vi "MeasurementControl - Main.vi"() -> ()   [LabVIEW 2014]
doc: "This VI provides control and an interface the various instruments used to collect data in the CLTC measurement lab. It is built based on the queued message handler template. It functions by sending commands to the queues of the various instrument VIs that are dynamically launched for a particular test."
uses:
  controls/Tab Control.ctl
  controls/Instrument Control Switches.ctl
  Timing and Stabilization/Stabilization.ctl
  avantesSpectrometer/Acquisition/Sphere Indicator.ctl
  controls/Time Left.ctl
  controls/Analyzer Choice.ctl
  avantesSpectrometer/Settings/Measurement Type.ctl
  avantesSpectrometer/Acquisition/AvaSpec Color Parameters.ctl
  Support/MeasurementControl Message Queue Folder/MeasurementControl Message Queue.lvlib
  avantesSpectrometer/AvaSpec.lvlib
  Launcher/Instrument Launcher.lvlib
  Timing and Stabilization/Timing and Stabilization.lvlib
  Support/Measurement Control User Event - Stop.lvlib
  avantesSpectrometer/Acquisition/AvaSpec Acquisition.lvlib
  Metadata/Metadata.lvlib
panel:
  in  "Start LM-79\nInsulated Sphere":bool
  in  "Start LM-79\nNaked Sphere":bool
  in  "Set Metadata":bool
  in  "Auto toggle tab":bool=TRUE
  in  "Analyzer Choice":T1
  in  "Instrument Control \nSwitches":T2
  in  "Exit":bool
  out "Status":string
  in  "Tab Control":T3
  out "Naked Sphere Stabilization Data":T4={"Stabilization waveform"={"t0"=timestamp(0 s since 1904-01-01), "dt"=50.0, "Y"=[10.0, 9.0, 8.75, 8.5, 8.25, 8.125, 8.06, 8.03, 8.015, 8.0, 8.0, 8.0]}, "Variation"=0.0, "Stabilized"=FALSE, "Threshold"=0.0, "time to stabilize"=0.0, "3 points"=[], "Sphere Indicator"=enum."Naked Sphere"}
  out "Insulated Sphere Stabilization Data":T4={"Stabilization waveform"={"t0"=timestamp(0 s since 1904-01-01), "dt"=50.0, "Y"=[10.0, 9.0, 8.75, 8.5, 8.25, 8.125, 8.06, 8.03, 8.015, 8.0, 8.0, 8.0]}, "Variation"=0.0, "Stabilized"=FALSE, "Threshold"=0.0, "time to stabilize"=0.0, "3 points"=[], "Sphere Indicator"=enum."Naked Sphere"}
  out "Time Left":T6 {"Naked Sphere Time Left" format="%#_2g"; "Insulated Sphere Time Left" format="%#_2g"}
  # "Start LM-79 \nStabilization"
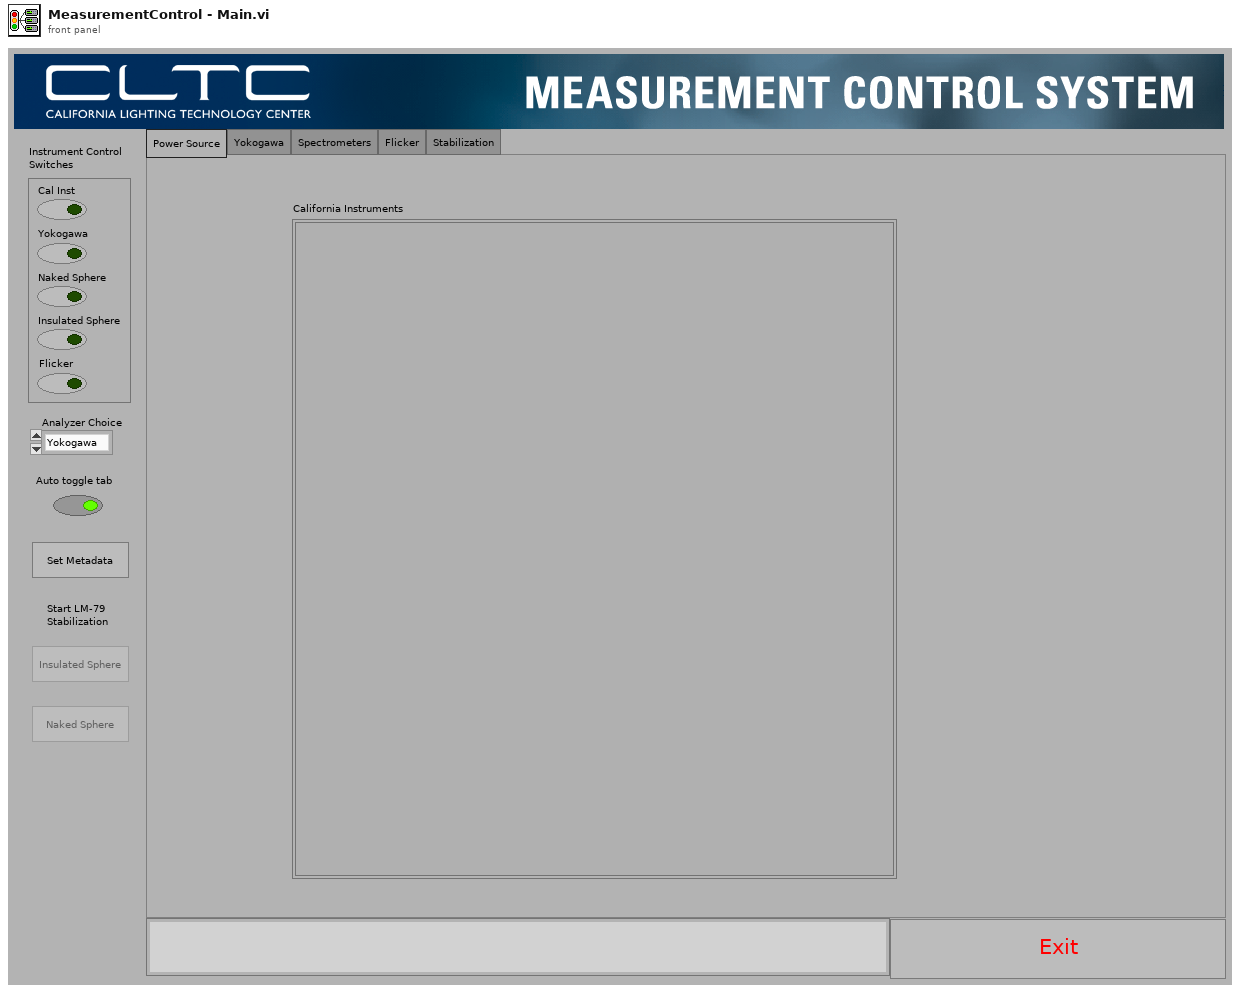
[diagram p1: front panel]
types:
  T1 = typedef "Analyzer Choice.ctl" = enum16{"Yokogawa", "Cal Inst"}
  T2 = typedef "Instrument Control Switches.ctl" = cluster{"Cal Inst":bool, "Yokogawa":bool, "Naked Sphere":bool, "Insulated Sphere":bool, "Flicker":bool}
  T3 = typedef "Tab Control.ctl" = enum32{"Power Source", "Yokogawa", "Spectrometers", "Flicker", "Stabilization"}
  T4 = typedef "Timing and Stabilization.lvlib/Stabilization.ctl" = cluster{"Stabilization waveform":waveform(dbl), "Variation":dbl, "Stabilized":bool, "Threshold":dbl, "time to stabilize":dbl, "3 points":dbl[], "Sphere Indicator":T5}
  T5 = typedef "AvaSpec.lvlib/Sphere Indicator.ctl" = enum16{"Naked Sphere", "Insulated Sphere"}
  T6 = typedef "Time Left.ctl" = cluster{"Naked Sphere Time Left":dbl, "Insulated Sphere Time Left":dbl}
  T7 = typedef "MeasurementControl Message Queue.lvlib/All Message Queues.ctl" = cluster{"Master":refnum<queue>, "UI":refnum<queue>, "Stabilization":refnum<queue>, "Timing":refnum<queue>}
  T8 = typedef "AvaSpec.lvlib/AvaSpec Acquisition.lvlib/Measurement Type.ctl" = enum16{"Normal", "Calibration", "Dark"}
  T9 = enum8{"Enabled", "Disabled", "Disabled and Grayed Out"}
  T10 = typedef "Metadata Cluster.ctl" = cluster{"Naked Sphere Metadata":string[][], "Insulated Sphere Metadata":string[][], "Output Path":path}
  T11 = typedef "AvaSpec.lvlib/AvaSpec Color Parameters.ctl" = cluster{"Power Spectral Distribution":cluster{"X":dbl, "Y":dbl}[], "Color Values":cluster{"luminousFlux":dbl, "CCT":dbl, "CRI":dbl, "u'":dbl, "v'":dbl, "Duv":dbl}, "R values":dbl[], "Chromaticity \nCoordinates":cluster{"x":dbl, "y":dbl, "z":dbl, "u":dbl, "v":dbl}, "Tristimulus \nValues":cluster{"X":dbl, "Y":dbl, "Z":dbl}, "Time Stamp":timestamp, "Temperature":dbl, "Integration Time":dbl, "Sphere Indicator":T5}
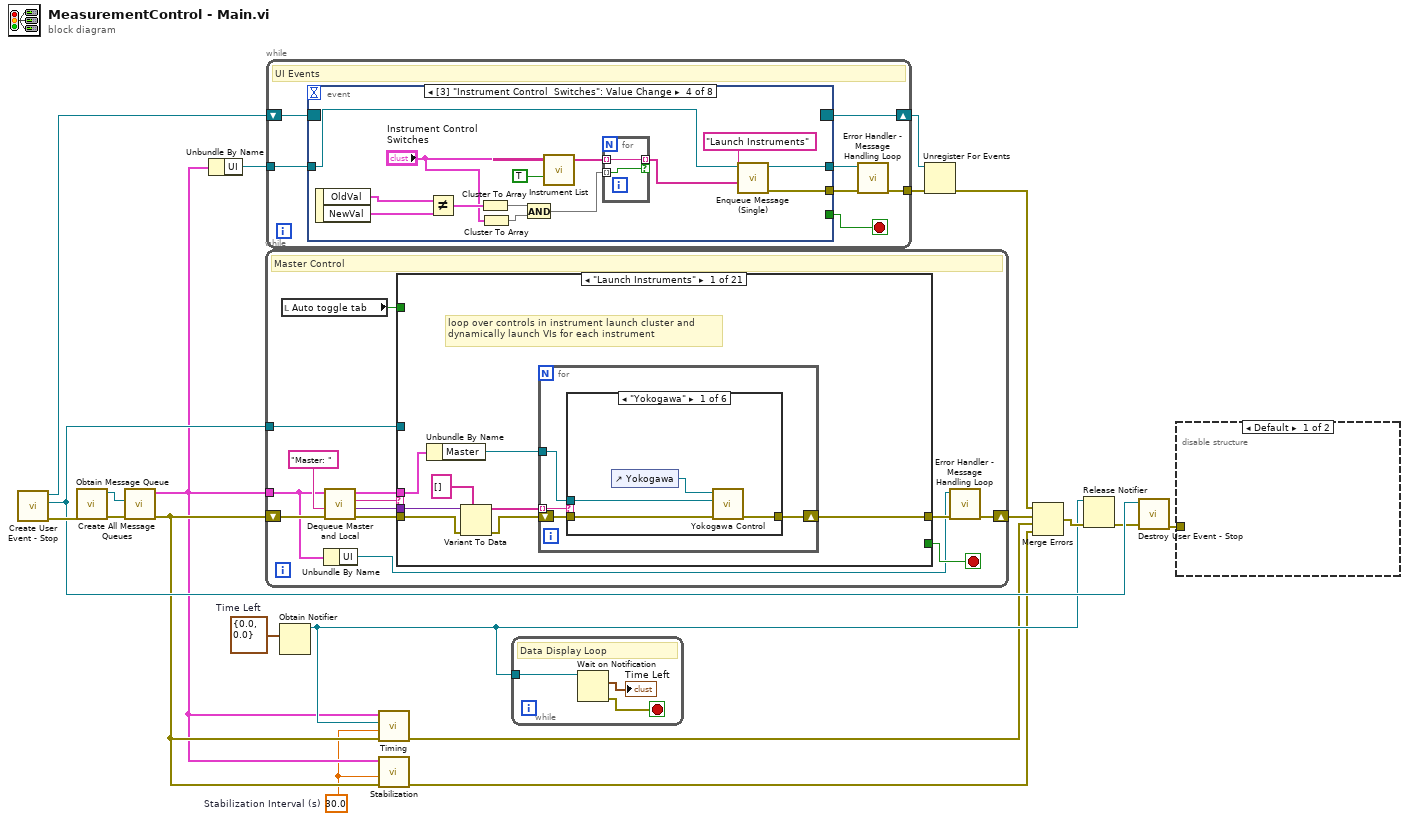
[diagram p0: block diagram]
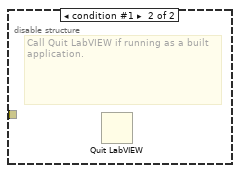
[diagram p2: hidden frame]
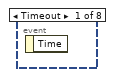
[diagram p3: hidden frame]
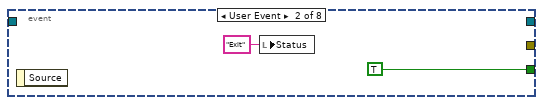
[diagram p4: hidden frame]
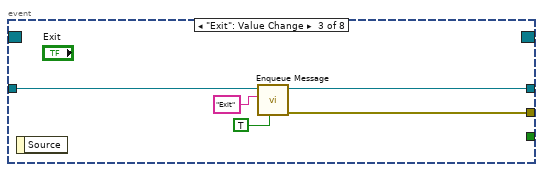
[diagram p5: hidden frame]
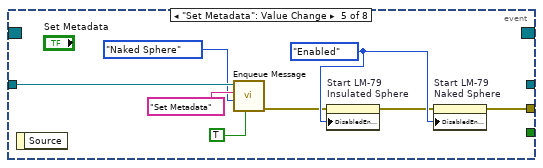
[diagram p6: hidden frame]
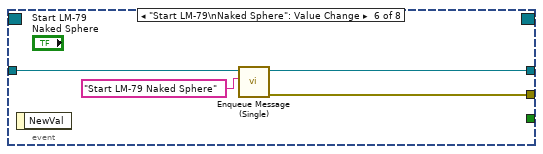
[diagram p7: hidden frame]
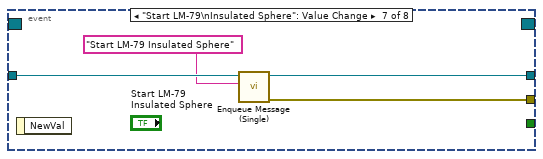
[diagram p8: hidden frame]
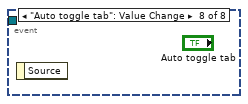
[diagram p9: hidden frame]
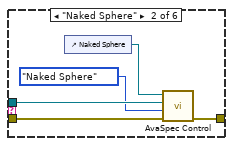
[diagram p10: hidden frame]
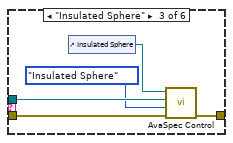
[diagram p11: hidden frame]
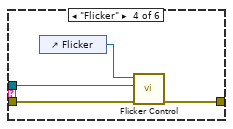
[diagram p12: hidden frame]
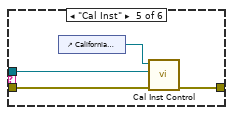
[diagram p13: hidden frame]
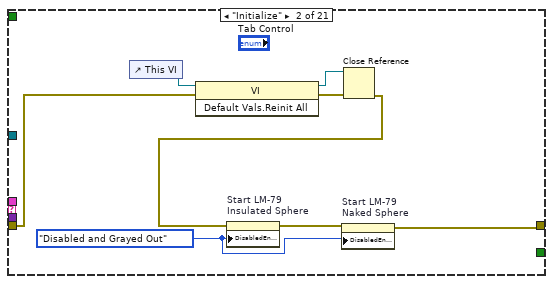
[diagram p15: hidden frame]
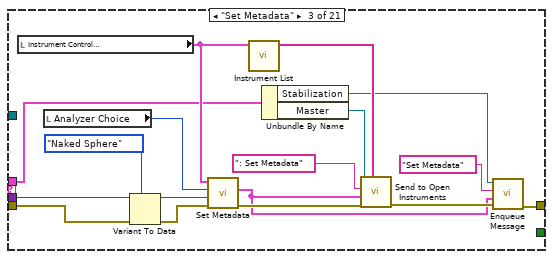
[diagram p16: hidden frame]
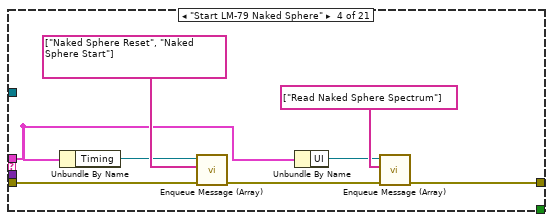
[diagram p17: hidden frame]
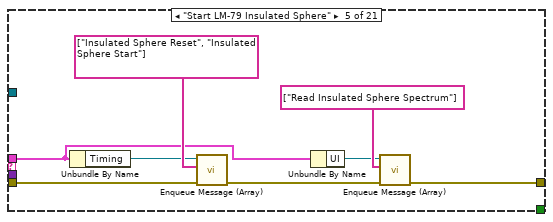
[diagram p18: hidden frame]
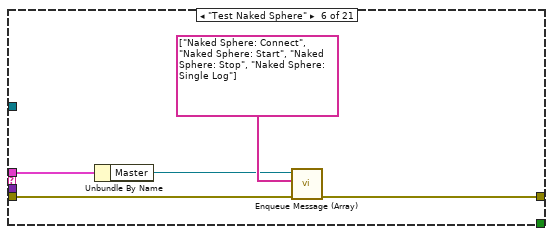
[diagram p19: hidden frame]
diagram:
  w10 = T6 {"Naked Sphere Time Left"=0.0, "Insulated Sphere Time Left"=0.0}  # Time Left
  w1 = 30.0  # Stabilization Interval (s)
  n1 = call "Create User Event - Stop.vi"() -> ("error out"=w18:errorcluster, "User Event - Stop"=w11:refnum<user-event>, "Stop Event Registration Refnum"=w14:refnum<event-registration>)  [unwired: 9 in]
  n2 = call "Obtain Message Queue.vi"("error in (no error)"=w18) -> ("error out"=w19:errorcluster, "Message Queue"=w20:refnum<queue>)  [unwired: 9 in]
  n3 = call "Create All Message Queues.vi"("error in (no error)"=w19, "Master Queue In"=w20) -> ("error out"=w7:errorcluster, "Message Queues out"=w2:T7)  [unwired: 8 in]
  n4 = Unbundle By Name(w2) -> ("UI"=w3:refnum<queue>)
  n5 = while {
    shift-right: [w25] -> w17
    shift-left: w7 -> [w32]
    tunnel: w2 -> [w22]
    tunnel: w11 -> [w28]
    stop <- w29 stop-if-true
    # "Master Control"
    n6 = local read "Auto toggle tab"() -> (w27:bool)
    n7 = Unbundle By Name(w22) -> ("UI"=w21:refnum<queue>)
    n8 = call "Dequeue Master and Local.vi"("error in (no error)"=w32, "Instrument Name"="Master: ", "Message Queues In"=w22) -> ("error out"=w33:errorcluster, "Message Data"=w31:variant, "Message"=w24:string, "Message Queues out"=w23:T7)  [unwired: 5 in]
    n9 = case shown="\"Launch Instruments\"" w24 {
      tunnel: w33 -> [w41 w70 w92 w97 w105 w112 w115 w132 w151 w154 w161 w181 w188 w201 w207 w226 w228 w232 w235 w253 _]
      tunnel: w31 -> [w40 _ w90 _ _ _ _ _ _ _ w159 _ _ w202 w208 w227 _ w230 _ _ w266]
      tunnel: [w39 w75 w82 w100 w108 w113 w115 w121 w141 w154 w164 w186 w188 w200 w206 w216 w228 w231 w235 w246 w260] -> w26
      tunnel: w23 -> [w35 _ w79 w95 w103 w111 _ w117 w135 _ w156 w184 _ w192 _ w213 _ _ _ w238 w259]
      tunnel: [_ _ _ _ _ _ _ _ _ _ _ _ _ _ _ _ _ _ _ TRUE _] -> w29
      tunnel: w28 -> [_ _ _ _ _ _ _ _ _ _ _ _ _ _ _ _ _ _ _ w248 _]
      tunnel: w27 -> [_ _ _ _ _ _ _ w124 w143 _ w162 w185 _ w194 _ _ _ _ _ _ _]
      frame "Launch Instruments" {
        # "loop over controls in instrument launch cluster and \ndynamically launch VIs for each instrument"
        n10 = Unbundle By Name(w35) -> ("Master"=w34:refnum<queue>)
        n11 = Variant To Data(error in=w41, type=string[] [], Variant=w40) -> (data=w37:string[], error out=w36:errorcluster)
        n12 = for {
          tunnel: w37 -> [w45] mode=indexing
          shift-right: [w42] -> w39
          shift-left: w36 -> [w44]
          tunnel: w34 -> [w43]
          n13 = case shown="\"Yokogawa\"" w45 {
            tunnel: w43 -> [w48 w52 w58 w62 w67 _]
            tunnel: [w47 w54 w57 w60 w65 w68] -> w42
            tunnel: w44 -> [w46 w51 w56 w61 w64 w68]
            frame "Yokogawa" {
              n14 = control-ref of="Yokogawa"() -> (w49:refnum<vi>)
              n15 = call "Yokogawa Control.vi"("error in (no error)"=w46, "Master"=w48, "reference"=w49) -> ("error out"=w47:errorcluster)  [unwired: 8 in]
            }
            frame "Naked Sphere" {
              n16 = control-ref of="Naked Sphere"() -> (w53:refnum<vi>)
              n17 = call "AvaSpec Control.vi"("error in (no error)"=w51, "Sphere Indicator"=Sphere_Indicator."Naked Sphere", "Master"=w52, "Subpanel ref"=w53) -> ("error out"=w54:errorcluster)  [unwired: 7 in]
            }
            frame "Insulated Sphere" {
              n18 = control-ref of="Insulated Sphere"() -> (w59:refnum<vi>)
              n19 = call "AvaSpec Control.vi"("error in (no error)"=w56, "Sphere Indicator"=Sphere_Indicator."Insulated Sphere", "Master"=w58, "Subpanel ref"=w59) -> ("error out"=w57:errorcluster)  [unwired: 7 in]
            }
            frame "Flicker" {
              n20 = control-ref of="Flicker"() -> (w63:refnum<vi>)
              n21 = call "Flicker Control.vi"("error in (no error)"=w61, "Master"=w62, "Sub Panel ref"=w63) -> ("error out"=w60:errorcluster)  [unwired: 8 in]
            }
            frame "Cal Inst" {
              n22 = control-ref of="California Instruments"() -> (w66:refnum<vi>)
              n23 = call "Cal Inst Control.vi"("error in (no error)"=w64, "Master"=w67, "Sub Panel ref"=w66) -> ("error out"=w65:errorcluster)  [unwired: 8 in]
            }
            frame Default {
            }
          }
        }
      }
      frame "Initialize" {
        w74 = T9."Disabled and Grayed Out" ("Disabled")
        n24 = control-ref of="This VI"() -> (w73:refnum<vi>)
        n25 = invoke class="VI" method="Default Vals.Reinit All"(reference=w73, error in=w70) -> (reference out=w72:refnum<vi>, error out=w71:errorcluster)  [unwired: 1 in, 1 out]
        n26 = Close Reference(reference=w72, error in (no error)=w71) -> (error out=w69:errorcluster)
        n27 = property on="Start LM-79\nInsulated Sphere" class="Bool"(error in=w69, "DisabledEnum"=w74) -> (error out=w76:errorcluster)  [unwired: 1 in, 1 out]
        n28 = property on="Start LM-79\nNaked Sphere" class="Bool"(error in=w76, "DisabledEnum"=w74) -> (error out=w75:errorcluster)  [unwired: 1 in, 1 out]
      }
      frame "Set Metadata" {
        n29 = local read "Instrument Control \nSwitches"() -> (w87:T2)
        n30 = local read "Analyzer Choice"() -> (w93:T1)
        n31 = Variant To Data(error in=w92, type=Sphere_Indicator."Naked Sphere" ("Sphere Indicator"), Variant=w90) -> (data=w91:T5, error out=w88:errorcluster)
        n32 = call "Set Metadata.vi"("error in (no error)"=w88, "Sphere Indicator"=w91, "Analyzer Choice"=w93, "Instrument Control \nSwitches"=w87) -> ("error out"=w86:errorcluster, "Metadata Cluster Out"=w80:T10)  [unwired: 6 in]
        n33 = call "Instrument List.vi"("Instrument Control Switches"=w87) -> ("Instrument Names"=w85:string[])  [unwired: 10 in]
        n34 = Unbundle By Name(w79) -> ("Stabilization"=w77:refnum<queue>, "Master"=w78:refnum<queue>)
        n35 = call "Send to Open Instruments.vi"("Instrument Names"=w85, "error in (no error)"=w86, "Message Data"=w80, "Command"=": Set Metadata", "Master"=w78) -> ("error out"=w83:errorcluster)  [unwired: 6 in]
        n36 = call-poly "Enqueue Message.vi"("error in (no error)"=w83, "Message Data"=w80, "Message"="Set Metadata", "Message Queue"=w77) -> ("error out"=w82:errorcluster)  [unwired: 6 in, 1 out]
      }
      frame "Start LM-79 Naked Sphere" {
        n37 = Unbundle By Name(w95) -> ("Timing"=w94:refnum<queue>)
        n38 = call "Enqueue Message (Array).vi"("error in (no error)"=w97, "Message Array"=string[] ["Naked Sphere Reset", "Naked Sphere Start"], "Message Queue"=w94) -> ("error out"=w99:errorcluster)  [unwired: 7 in, 1 out]
        n39 = Unbundle By Name(w95) -> ("UI"=w96:refnum<queue>)
        n40 = call "Enqueue Message (Array).vi"("error in (no error)"=w99, "Message Array"=string[] ["Read Naked Sphere Spectrum"], "Message Queue"=w96) -> ("error out"=w100:errorcluster)  [unwired: 7 in, 1 out]
      }
      frame "Start LM-79 Insulated Sphere" {
        n41 = Unbundle By Name(w103) -> ("Timing"=w102:refnum<queue>)
        n42 = call "Enqueue Message (Array).vi"("error in (no error)"=w105, "Message Array"=string[] ["Insulated Sphere Reset", "Insulated Sphere Start"], "Message Queue"=w102) -> ("error out"=w107:errorcluster)  [unwired: 7 in, 1 out]
        n43 = Unbundle By Name(w103) -> ("UI"=w104:refnum<queue>)
        n44 = call "Enqueue Message (Array).vi"("error in (no error)"=w107, "Message Array"=string[] ["Read Insulated Sphere Spectrum"], "Message Queue"=w104) -> ("error out"=w108:errorcluster)  [unwired: 7 in, 1 out]
      }
      frame "Test Naked Sphere" {
        n45 = Unbundle By Name(w111) -> ("Master"=w110:refnum<queue>)
        n46 = call "Enqueue Message (Array).vi"("error in (no error)"=w112, "Message Array"=string[] ["Naked Sphere: Connect", "Naked Sphere: Start", "Naked Sphere: Stop", "Naked Sphere: Single Log"], "Message Queue"=w110) -> ("error out"=w113:errorcluster)  [unwired: 7 in, 1 out]
      }
      frame "-----------Spectrometers-----------" {
      }
      frame "Read Naked Sphere Spectrum" {
        n47 = case shown="True" w124 {
          frame False {
          }
          frame True {
            n48 = local write "Tab Control"(Tab_Control."Spectrometers" ("Tab Control")) -> ()
          }
        }
        n49 = Unbundle By Name(w117) -> ("UI"=w116:refnum<queue>)
        n50 = call-poly "Enqueue Message.vi"("error in (no error)"=w132, "Message Data"="Read Naked Sphere Spectrum " ("Message"), "Message"="Update Status", "Message Queue"=w116) -> ("error out"=w128:errorcluster)  [unwired: 6 in, 1 out]
        n51 = Unbundle By Name(w117) -> ("Master"=w118:refnum<queue>)
        n52 = call-poly "Enqueue Message.vi"("error in (no error)"=w128, "Message Data"=Measurement_Type."Normal" ("Measurement Type In 2"), "Message"="Naked Sphere: Update Measurement Type", "Message Queue"=w118) -> ("error out"=w127:errorcluster, "dup Message Queue"=w129:refnum<queue>)  [unwired: 6 in]
        n53 = call "Enqueue Message (Array).vi"("error in (no error)"=w127, "Message Array"=string[] ["Naked Sphere: Connect", "Naked Sphere: Start"], "Message Queue"=w129) -> ("error out"=w122:errorcluster, "dup Message Queue"=w123:refnum<queue>)  [unwired: 7 in]
        n54 = call-poly "Enqueue Message.vi"("error in (no error)"=w122, "Message Data"=TRUE, "Message"="Naked Sphere: Save Data", "Message Queue"=w123) -> ("error out"=w121:errorcluster)  [unwired: 6 in, 1 out]
      }
      frame "Read Insulated Sphere Spectrum" {
        n55 = case shown="True" w143 {
          frame False {
          }
          frame True {
            n56 = local write "Tab Control"(Tab_Control."Spectrometers" ("Tab Control")) -> ()
          }
        }
        n57 = Unbundle By Name(w135) -> ("UI"=w136:refnum<queue>)
        n58 = call-poly "Enqueue Message.vi"("error in (no error)"=w151, "Message Data"="Read Insulated Sphere Spectrum " ("Message"), "Message"="Update Status", "Message Queue"=w136) -> ("error out"=w147:errorcluster)  [unwired: 6 in, 1 out]
        n59 = Unbundle By Name(w135) -> ("Master"=w137:refnum<queue>)
        n60 = call-poly "Enqueue Message.vi"("error in (no error)"=w147, "Message Data"=Measurement_Type."Normal" ("Measurement Type In 2"), "Message"="Insulated Sphere: Update Measurement Type", "Message Queue"=w137) -> ("error out"=w146:errorcluster, "dup Message Queue"=w148:refnum<queue>)  [unwired: 6 in]
        n61 = call "Enqueue Message (Array).vi"("error in (no error)"=w146, "Message Array"=string[] ["Insulated Sphere: Connect", "Insulated Sphere: Start"], "Message Queue"=w148) -> ("error out"=w142:errorcluster, "dup Message Queue"=w140:refnum<queue>)  [unwired: 7 in]
        n62 = call-poly "Enqueue Message.vi"("error in (no error)"=w142, "Message Data"=TRUE, "Message"="Insulated Sphere: Save Data", "Message Queue"=w140) -> ("error out"=w141:errorcluster)  [unwired: 6 in, 1 out]
      }
      frame "---------Electrical & Flicker---------" {
      }
      frame "Take Electrical Measurements" {
        n63 = case shown="True" w162 {
          tunnel: "Analyzer Choice" -> [_ w165]
          frame False {
          }
          frame True {
            n64 = case shown="\"Cal Inst\"" w165 {
              tunnel: [Tab_Control."Yokogawa" ("Tab Control") Tab_Control."Power Source" ("Tab Control")] -> w166
              frame "Yokogawa", Default {
              }
              frame "Cal Inst" {
              }
            }
            n65 = local write "Tab Control"(w166) -> ()
          }
        }
        n66 = Variant To Data(error in=w161, type=Sphere_Indicator."Naked Sphere" ("Sphere Indicator"), Variant=w159) -> (data=w157:T5, error out=w160:errorcluster)
        n67 = Unbundle By Name(w156) -> ("Master"=w155:refnum<queue>)
        n68 = case shown="\"Yokogawa\", Default" "Analyzer Choice" {
          tunnel: w155 -> [w173 w180]
          tunnel: w160 -> [w176 w179]
          tunnel: [w174 w178] -> w164
          tunnel: w157 -> [w169 _]
          frame "Yokogawa", Default {
            n69 = call-poly "Enqueue Message.vi"("error in (no error)"=w176, "Message"="Yokogawa: Start", "Message Queue"=w173) -> ("error out"=w175:errorcluster, "dup Message Queue"=w172:refnum<queue>)  [unwired: 7 in]
            n70 = call-poly "Enqueue Message.vi"("error in (no error)"=w175, "Message Data"=w169, "Message"="Yokogawa: Save Data", "Message Queue"=w172) -> ("error out"=w174:errorcluster)  [unwired: 6 in, 1 out]
          }
          frame "Cal Inst" {
            n71 = call "Enqueue Message (Array).vi"("error in (no error)"=w179, "Message Array"=string[] ["Cal Inst: Start Acquisition", "Cal Inst: Save Data"], "Message Queue"=w180) -> ("error out"=w178:errorcluster)  [unwired: 7 in, 1 out]
          }
        }
      }
      frame "Take Flicker Measurements" {
        n72 = case shown="True" w185 {
          frame False {
          }
          frame True {
            n73 = local write "Tab Control"(Tab_Control."Flicker" ("Tab Control")) -> ()
          }
        }
        n74 = Unbundle By Name(w184) -> ("Master"=w183:refnum<queue>)
        n75 = call "Enqueue Message (Array).vi"("error in (no error)"=w181, "Message Array"=string[] ["Flicker: Start Acquisition", "Flicker: Save Data"], "Message Queue"=w183) -> ("error out"=w186:errorcluster)  [unwired: 7 in, 1 out]
      }
      frame "-------------Stabilization------------" {
      }
      frame "Check for Stabilization" {
        w198 = T11 {"Power Spectral Distribution"=[], "Color Values"={"luminousFlux"=0.0, "CCT"=0.0, "CRI"=0.0, "u'"=0.0, "v'"=0.0, "Duv"=0.0}, "R values"=[], "Chromaticity \nCoordinates"={"x"=0.0, "y"=0.0, "z"=0.0, "u"=0.0, "v"=0.0}, "Tristimulus \nValues"={"X"=0.0, "Y"=0.0, "Z"=0.0}, "Time Stamp"=timestamp(0 s since 1904-01-01), "Temperature"=0.0, "Integration Time"=0.0, "Sphere Indicator"=enum."Naked Sphere"}  # Color Parameters
        n76 = case shown="True" w194 {
          frame False {
          }
          frame True {
            n77 = local write "Tab Control"(Tab_Control."Stabilization" ("Tab Control")) -> ()
          }
        }
        n78 = Variant To Data(error in=w201, type=w198, Variant=w202) -> (data=w199:T11, error out=w190:errorcluster)
        n79 = call "Stabilization status update.vi"("Color Parameters"=w199) -> ("luminousFlux"=w197:dbl, "Status String"=w195:string)  [unwired: 9 in]
        n80 = Unbundle By Name(w192) -> ("UI"=w191:refnum<queue>)
        n81 = call-poly "Enqueue Message.vi"("error in (no error)"=w190, "Message Data"=w195, "Message"="Update Status", "Message Queue"=w191) -> ("error out"=w189:errorcluster)  [unwired: 6 in, 1 out]
        n82 = Unbundle By Name(w192) -> ("Stabilization"=w193:refnum<queue>)
        n83 = call-poly "Enqueue Message.vi"("error in (no error)"=w189, "Message Data"=w197, "Message"=w195, "Message Queue"=w193) -> ("error out"=w200:errorcluster)  [unwired: 6 in, 1 out]
      }
      frame "Update Stabilization" {
        n84 = Variant To Data(error in=w207, type=T4 {"Stabilization waveform"={"t0"=timestamp(0 s since 1904-01-01), "dt"=50.0, "Y"=[10.0, 9.0, 8.75, 8.5, 8.25, 8.125, 8.06, 8.03, 8.015, 8.0, 8.0, 8.0]}, "Variation"=0.0, "Stabilized"=FALSE, "Threshold"=0.0, "time to stabilize"=0.0, "3 points"=[], "Sphere Indicator"=enum."Naked Sphere"} ("Stabilization Data"), Variant=w208) -> (data=w205:T4, error out=w206:errorcluster)
        n85 = Unbundle By Name(w205) -> ("Sphere Indicator"=w204:T5)
        n86 = case shown="\"Naked Sphere\", Default" w204 {
          tunnel: w205 -> [w210 w211]
          frame "Naked Sphere", Default {
            "Naked Sphere Stabilization Data" <- w210
          }
          frame "Insulated Sphere" {
            "Insulated Sphere Stabilization Data" <- w211
          }
        }
      }
      frame "Stabilization Complete" {
        n87 = Unbundle By Name(w213) -> ("UI"=w212:refnum<queue>)
        n88 = Variant To Data(error in=w226, type=Sphere_Indicator."Naked Sphere" ("Sphere Indicator"), Variant=w227) -> (data=w221:T5, error out=w224:errorcluster)
        n89 = Build Array(w221) -> (w222:T5[])
        n90 = call "Enqueue Message (Array).vi"("error in (no error)"=w224, "Message Data Array"=w222, "Message Array"=string[] ["Take Electrical Measurements", "Take Flicker Measurements"], "Message Queue"=w212) -> ("error out"=w218:errorcluster, "dup Message Queue"=w217:refnum<queue>)  [unwired: 6 in]
        n91 = Format Into String(w221) -> (resulting string=w220:string)  [unwired: 3 in, 1 out]
        n92 = Concatenate Strings(w220, " Electrical Measurements") -> (w215:string)
        n93 = call-poly "Enqueue Message.vi"("error in (no error)"=w218, "Message Data"=w215, "Message"="Update Status", "Message Queue"=w217) -> ("error out"=w216:errorcluster)  [unwired: 6 in, 1 out]
      }
      frame "----------------Misc-----------------" {
      }
      frame "Update Status" {
        n94 = Variant To Data(error in=w232, type="", Variant=w230) -> (data=→"Status":string, error out=w231:errorcluster)
      }
      frame "Ignore Message", Default {
        n95 = Wait (ms)(milliseconds to wait=u32 500) -> ()  [unwired: 1 out]
      }
      frame "Exit" {
        n96 = Unbundle By Name(w238) -> ("Master"=w236:refnum<queue>, "UI"=w237:refnum<queue>)
        n97 = local read "Instrument Control \nSwitches"() -> (w240:T2)
        n98 = call "Fire User Event - Stop.vi"("User Event - Stop"=w248) -> ("error out"=w245:errorcluster)  [unwired: 10 in]
        n99 = Release Queue(queue=w237, error in (no error)=w253) -> (error out=w243:errorcluster)  [unwired: 1 in, 2 out]
        n100 = call "Instrument List.vi"("Instrument Control Switches"=w240) -> ("Instrument Names"=w239:string[])  [unwired: 10 in]
        n101 = Cluster To Array(cluster=w238) -> (array=w251:refnum<queue>[])
        n102 = call "Send to Open Instruments.vi"("Instrument Names"=w239, "error in (no error)"=w243, "Command"=": Exit", "Master"=w236) -> ("error out"=w242:errorcluster)  [unwired: 7 in]
        n103 = Delete From Array(array=w251, length=2, index=0) -> (array with subset deleted=w249:refnum<queue>[])  [unwired: 1 out]
        n104 = for {
          tunnel: w249 -> [w257] mode=indexing
          shift-right: [w255] -> w247
          shift-left: w242 -> [w254]
          # "Exit all Modules"
          n105 = call "Enqueue Message (Single).vi"("error in (no error)"=w254, "Message"="Exit", "Message Queue"=w257) -> ("error out"=w255:errorcluster)  [unwired: 7 in, 1 out]
        }
        n106 = Merge Errors(w245, w247) -> (w246:errorcluster)
      }
      frame "Error" {
        n107 = Unbundle By Name(w259) -> ("UI"=w258:refnum<queue>)
        n108 = Variant To Data(type=errorcluster {"status"=FALSE, "code"=0, "source"=""} ("error constant"), Variant=w266) -> (data=w261:errorcluster, error out=w263:errorcluster)  [unwired: 1 in]
        n109 = disable-structure shown="Disabled" {
          frame Disabled {
            n110 = call "Custom Error Handler.vi"() -> ()  [unwired: 11 in, 1 out]
          }
          frame Enabled {
          }
        }
        n111 = call <vilib>:"Simple Error Handler.vi"("error in (no error)"=w261) -> ()  [unwired: 4 in, 5 out]
        n112 = call-poly "Enqueue Message.vi"("Priority Message? (F)"=TRUE, "Message"="Exit", "Message Queue"=w258) -> ("error out"=w262:errorcluster)  [unwired: 7 in, 1 out]
        n113 = Merge Errors(w262, w263) -> (w260:errorcluster)
      }
    }
    n114 = call "Error Handler - Message Handling Loop.vi"("error in (no error)"=w26, "Message Queue"=w21) -> ("dup error in"=w25:errorcluster)  [unwired: 8 in, 1 out]
  }
  n115 = while {
    tunnel: w3 -> [w274]
    shift-right: [w273] -> w15
    shift-left: w14 -> [w272]
    tunnel: [w269] -> w13
    stop <- w271 stop-if-true
    # "UI Events"
    n116 = event shown="[3] \"Instrument Control  Switches\": Value Change" {
      selector: w272 -> [_ _ _ _ _ _ _ _]
      dyn-events: [_ _ _ _ _ _ _ _] -> w273
      timeout: _ -> [_ _ _ _ _ _ _ _]
      tunnel: w274 -> [_ _ w281 w293 w305 w309 w313 _]
      tunnel: [_ TRUE _ _ _ _ _ _] -> w271
      tunnel: [_ _ w279 w291 w299 w307 w310 _] -> w270
      tunnel: [_ _ w277 w286 _ w306 w311 _] -> w268
      event Timeout {
        n117 = event-data() -> ()  [unwired: 1 in, 1 out]
      }
      event User Event {
        n118 = event-data() -> ()  [unwired: 1 in, 1 out]
        n119 = local write "Status"("Exit" ("Status")) -> ()
      }
      event "Exit": Value Change {
        n120 = event-data() -> ()  [unwired: 1 in, 1 out]
        n121 = call-poly "Enqueue Message.vi"("Priority Message? (F)"=TRUE, "Message"="Exit", "Message Queue"=w281) -> ("error out"=w279:errorcluster, "dup Message Queue"=w277:refnum<queue>)  [unwired: 7 in]
      }
      event Value Change {
        n122 = event-data() -> ("OldVal"=w289:T2, "NewVal"=w288:T2)  [unwired: 1 in]
        n123 = Not Equal?(x=w289, y=w288) -> (x != y?=w295:T2)
        n124 = Cluster To Array(cluster=w295) -> (array=w284:bool[])
        n125 = Cluster To Array(cluster="Instrument Control \nSwitches") -> (array=w283:bool[])
        n126 = And(x=w284, y=w283) -> (x .and. y?=w282:bool[])
        n127 = call "Instrument List.vi"("All"=TRUE, "Instrument Control Switches"="Instrument Control \nSwitches") -> ("Instrument Names"=w294:string[])  [unwired: 9 in]
        n128 = for {
          tunnel: w282 -> [w296] mode=indexing
          tunnel: w294 -> [w297] mode=indexing
          tunnel: [w297] -> w292 mode=indexing if=w296
        }
        n129 = call "Enqueue Message (Single).vi"("Message Data"=w292, "Message"="Launch Instruments", "Message Queue"=w293) -> ("error out"=w291:errorcluster, "dup Message Queue"=w286:refnum<queue>)  [unwired: 7 in]
      }
      event "Set Metadata": Value Change {
        w301 = T9."Enabled" ("Disabled")
        n130 = event-data() -> ()  [unwired: 1 in, 1 out]
        n131 = call-poly "Enqueue Message.vi"("Priority Message? (F)"=TRUE, "Message Data"=Sphere_Indicator."Naked Sphere" ("Sphere Indicator"), "Message"="Set Metadata", "Message Queue"=w305) -> ("error out"=w298:errorcluster)  [unwired: 6 in, 1 out]
        n132 = property on="Start LM-79\nInsulated Sphere" class="Bool"(error in=w298, "DisabledEnum"=w301) -> (error out=w300:errorcluster)  [unwired: 1 in, 1 out]
        n133 = property on="Start LM-79\nNaked Sphere" class="Bool"(error in=w300, "DisabledEnum"=w301) -> (error out=w299:errorcluster)  [unwired: 1 in, 1 out]
      }
      event "Start LM-79\nNaked Sphere": Value Change {
        n134 = event-data() -> ()  [unwired: 1 in, 1 out]
        n135 = call "Enqueue Message (Single).vi"("Message"="Start LM-79 Naked Sphere", "Message Queue"=w309) -> ("error out"=w307:errorcluster, "dup Message Queue"=w306:refnum<queue>)  [unwired: 8 in]
      }
      event "Start LM-79\nInsulated Sphere": Value Change {
        n136 = event-data() -> ()  [unwired: 1 in, 1 out]
        n137 = call "Enqueue Message (Single).vi"("Message"="Start LM-79 Insulated Sphere", "Message Queue"=w313) -> ("error out"=w310:errorcluster, "dup Message Queue"=w311:refnum<queue>)  [unwired: 8 in]
      }
      event "Auto toggle tab": Value Change {
        n138 = event-data() -> ()  [unwired: 1 in, 1 out]
      }
    }
    n139 = call "Error Handler - Message Handling Loop.vi"("error in (no error)"=w270, "Message Queue"=w268) -> ("dup error in"=w269:errorcluster)  [unwired: 8 in, 1 out]
  }
  n140 = Obtain Notifier(notification data type=w10) -> (notifier out=w6:refnum<notifier>)  [unwired: 3 in, 2 out]
  n141 = call "Timing.vi"("error in"=w7, "Stabilization Interval (s)"=w1, "Time Left"=w6, "Message Queues out"=w2) -> ("error out"=w5:errorcluster)  [unwired: 7 in]
  n142 = call "Stabilization.vi"("error in (no error)"=w7, "Stabilization Interval (s)"=w1, "Message Queues out"=w2) -> ("error out"=w4:errorcluster)  [unwired: 8 in]
  n143 = while {
    tunnel: w6 -> [w314]
    stop <- w316 stop-if-true
    # "Data Display Loop"
    n144 = Wait on Notification(notifier=w314) -> (notification=→"Time Left":T6, error out=w316:errorcluster)  [unwired: 3 in, 2 out]
  }
  n145 = Unregister For Events(event registration refnum=w15, error in=w13) -> (error out=w16:errorcluster)
  n146 = Merge Errors(w16, w17, w5, w4) -> (w9:errorcluster)
  n147 = Release Notifier(notifier=w6, error in (no error)=w9) -> (error out=w8:errorcluster)  [unwired: 1 in, 2 out]
  n148 = call "Destroy User Event - Stop.vi"("error in (no error)"=w8, "User Event - Stop"=w11) -> ("error out"=w12:errorcluster)  [unwired: 9 in]
  n149 = disable-structure shown="Default" {
    disable-tunnel: w12 -> [_ _]
    frame condition #0 (active) {
    }
    frame condition #1 {
      # "Call Quit LabVIEW if running as a built application."
      n150 = Quit LabVIEW() -> ()  [unwired: 1 in]
    }
  }
